vi "SRV_Initialize All Motors Config Array.vi"(0 "All Motor Control Config":T1[](array[typedef]) {"Release Cmds"."Motor Control Commands Array"."Value" format="%02x"; "Release Cmds"."Motor Control Commands Array"."Register" format="%02x"; "Release Cmds"."Motor Control Commands Array"."I2C Address" format="%02x"; "Press Cmds"."Motor Control Commands Array"."Value" format="%02x"; "Press Cmds"."Motor Control Commands Array"."Register" format="%02x"; "Press Cmds"."Motor Control Commands Array"."I2C Address" format="%02x"}, 12 "Reset Icons to Blank? (F)":bool) -> (4 "All Motor Control Config out":T1[](array[typedef]) {"Release Cmds"."Motor Control Commands Array"."Value" format="%02x"; "Release Cmds"."Motor Control Commands Array"."Register" format="%02x"; "Release Cmds"."Motor Control Commands Array"."I2C Address" format="%02x"; "Press Cmds"."Motor Control Commands Array"."Value" format="%02x"; "Press Cmds"."Motor Control Commands Array"."Register" format="%02x"; "Press Cmds"."Motor Control Commands Array"."I2C Address" format="%02x"})   [LabVIEW 2014]
doc: "Author: Mike Schultz (LogicPD, Inc)"
uses:
  SRV_Motor Control Button Config.ctl
  SRV_Motor Legos-Servo.ctl
  SRV_Motor Control Commands Cluster.ctl
  SRV_Motor Control Command Config.ctl
  SRV_Motor Control Button Icons_FALSE.ctl
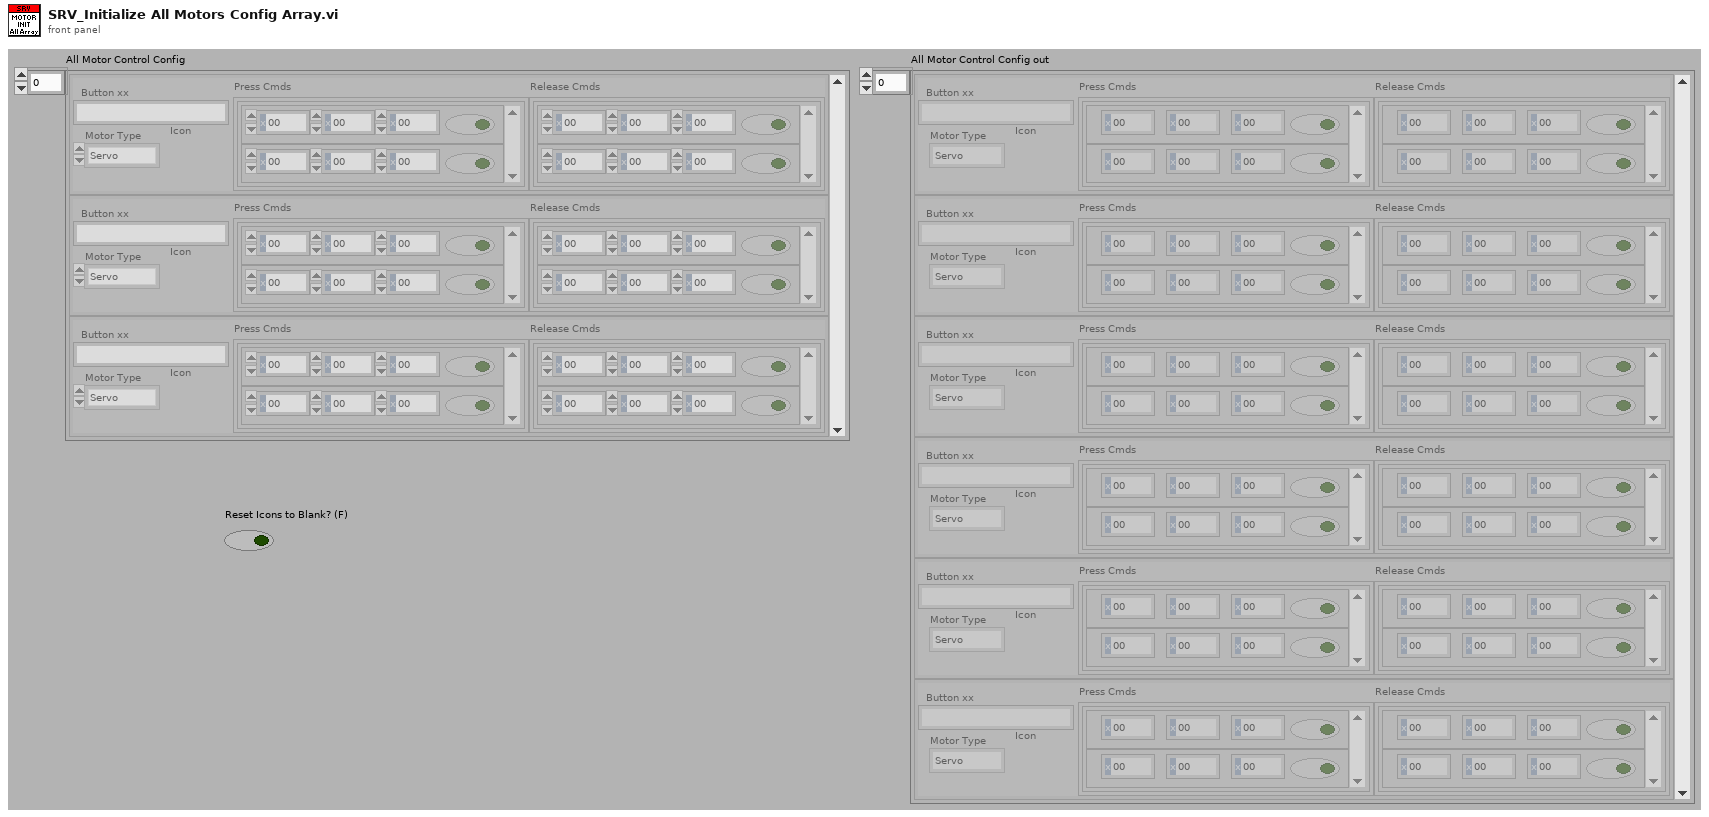
[diagram p1: front panel]
types:
  T1 = typedef "SRV_Motor Control Button Config.ctl" = cluster{"Button Name":string, "Button Label":string, "Motor Type":T2, "Press Cmds":T3, "Release Cmds":T3, "Icon":T5}
  T2 = typedef "SRV_Motor Legos-Servo.ctl" = enum16{"Servo", "Legos", "Shared Var"}
  T3 = typedef "SRV_Motor Control Commands Cluster.ctl" = cluster{"Motor Control Commands Array":T4[]}
  T4 = typedef "SRV_Motor Control Command Config.ctl" = cluster{"I2C Address":u8, "Register":u8, "Value":u8, "Active":bool}
  T5 = typedef "SRV_Motor Control Button Icons_FALSE.ctl" = u16
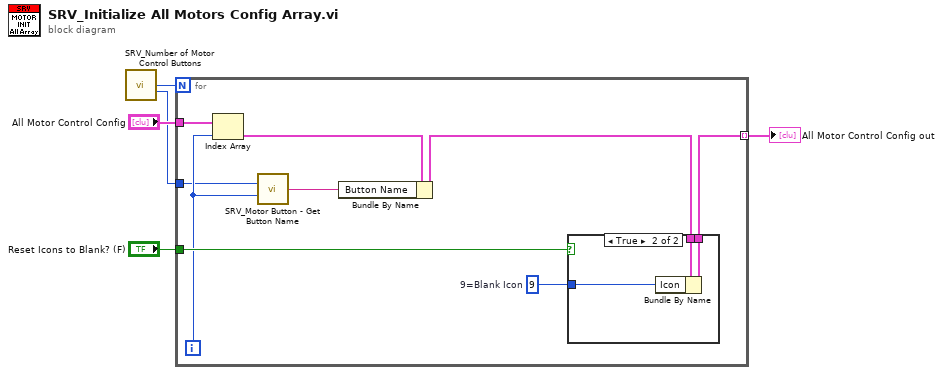
[diagram p0: block diagram]
diagram:
  n1 = call "SRV_Number of Motor Control Buttons.vi"() -> ("Number of Motor Control Buttons"=w3:i32, "Number of Columns"=w1:i32)  [unwired: 14 in]
  n2 = for {
    N: w3 -> [_]
    tunnel: "All Motor Control Config" -> [w14]
    tunnel: [w13] -> w4 mode=indexing
    tunnel: "Reset Icons to Blank? (F)" -> [w9]
    tunnel: w1 -> [w6]
    i -> [w7]
    w10 = T5 9  # 9=Blank Icon
    n3 = Index Array(array=w14, index=w7) -> (element=w12:T1)
    n4 = call "SRV_Motor Button - Get Button Name.vi"("Number of Columns"=w6, "Index"=w7) -> ("Button Name"=w8:string)  [unwired: 13 in]
    n5 = Bundle By Name(cluster=w12, "Button Name"=w8) -> (w11:T1)
    n6 = case shown="True" w9 {
      tunnel: w10 -> [_ w18]
      tunnel: w11 -> [w15 w17]
      tunnel: [w15 w16] -> w13
      frame False {
      }
      frame True {
        n7 = Bundle By Name(cluster=w17, "Icon"=w18) -> (w16:T1)
      }
    }
  }
  "All Motor Control Config out" <- w4
